vi "Config Scan Frequency.vi"(0 "VISA resource name":refnum<visa-resource-name>, 1 "Coupling (0)":i32 min=0 max=3, 2 "Floor (50 Hz)":dbl=50.0 min=50.0 max=20000.0, 3 "Ceiling (20000 Hz)":dbl=20000.0 min=50.0 max=20000.0, 4 "Method (discrete)":enum16{"discrete", "log10", "log2", "linear"}(ring), 5 "Method Value (-12)":dbl=-12.0 min=-19000.0 max=19000.0, 7 "error in":errorcluster) -> (20 "VISA resource name out":refnum<visa-resource-name>, 27 "error out":errorcluster)   [LabVIEW 2019, in "Andeen-Hagerling 2700(400 firmware).lvlib"]
doc: "Establishes the position of frequency scanning within the multidimensional parameter scanning system. Also sets the range of frequency used during scanning as well as the direction in which the frequency is changed each time a scan measurement is to be taken."
uses:
  Andeen-Hagerling 2700(400 firmware).lvlib
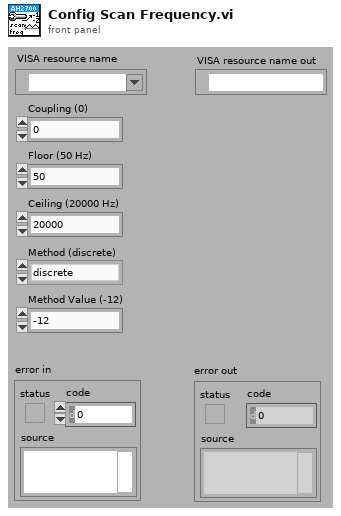
[diagram p1: front panel]
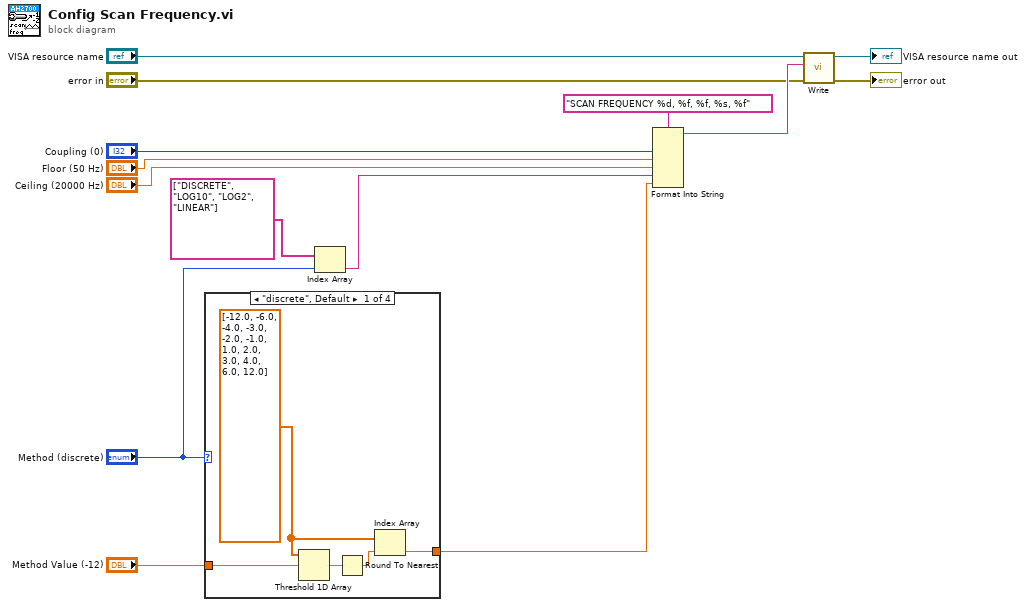
[diagram p0: block diagram]
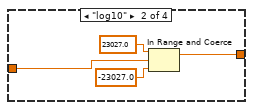
[diagram p2: hidden frame]
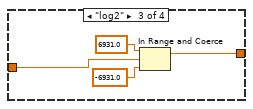
[diagram p3: hidden frame]
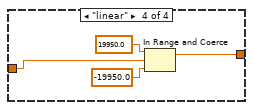
[diagram p4: hidden frame]
diagram:
  n1 = case shown="\"discrete\", Default" "Method (discrete)" {
    tunnel: "Method Value (-12)" -> [w16 w20 w24 w28]
    tunnel: [w15 w21 w25 w29] -> w1
    frame "discrete", Default {
      w17 = dbl[] [-12.0, -6.0, -4.0, -3.0, -2.0, -1.0, 1.0, 2.0, 3.0, 4.0, 6.0, 12.0]
      n2 = Threshold 1D Array(2:w16, 3:w17) -> (0:w19:dbl)  [unwired: 1 in]
      n3 = Round To Nearest(number=w19) -> (nearest integer value=w18:dbl)
      n4 = Index Array(array=w17, index=w18) -> (element=w15:dbl)
    }
    frame "log10" {
      n5 = In Range and Coerce(upper limit=23027.0, x=w20, lower limit=-23027.0) -> (coerced(x)=w21:dbl)  [unwired: 1 out]
    }
    frame "log2" {
      n6 = In Range and Coerce(upper limit=6931.0, x=w24, lower limit=-6931.0) -> (coerced(x)=w25:dbl)  [unwired: 1 out]
    }
    frame "linear" {
      n7 = In Range and Coerce(upper limit=19950.0, x=w28, lower limit=-19950.0) -> (coerced(x)=w29:dbl)  [unwired: 1 out]
    }
  }
  n8 = Index Array(array=string[] ["DISCRETE", "LOG10", "LOG2", "LINEAR"], index="Method (discrete)") -> (element=w2:string)
  n9 = Format Into String(format string="SCAN FREQUENCY %d, %f, %f, %s, %f", "Coupling (0)", "Floor (50 Hz)", "Ceiling (20000 Hz)", w2, w1) -> (resulting string=w14:string)  [unwired: 2 in, 1 out]
  n10 = call "Write.vi"("error in"="error in", "command"=w14, "VISA resource name"="VISA resource name") -> ("error out"=→"error out":errorcluster, "VISA resource name out"=→"VISA resource name out":refnum<visa-resource-name>)  [unwired: 7 in]
